vi "RudderToPoint.vi"(1 "Angle to Check":dbl) -> (8 "Goodness":dbl)   [LabVIEW 2012]
doc: "Takes in an angle to check, and returns a goodness value related to how close said angle is to the angle between the robot and the waypoint.\n\nTODO: Convert to using angle class"
uses:
  Sailbot Trunk/Software/2-Think/2 Typedefs/UTM Location.ctl
  Midbrain/Act/GoToWaypoint/RudderToPointEnum.ctl
  Utilities/Math/Angles/Angle/Angle.lvclass
panel:
  in  "Enum":T1
  in  "Robot Angle":dbl
  in  "Robot Location":T2 {"North" format="%#_10f"; "East" format="%#_8f"}
  in  "Waypoint":T2 {"North" format="%#_10f"; "East" format="%#_8f"}
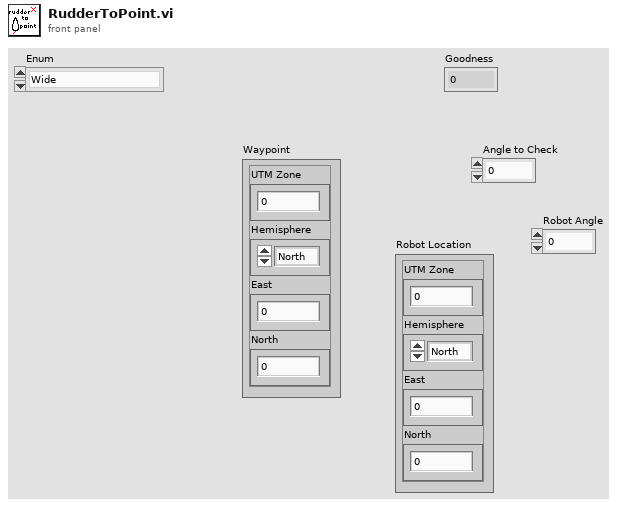
[diagram p1: front panel]
types:
  T1 = typedef "RudderToPointEnum.ctl" = enum16{"Wide", "Very Wide", "Conservative", "Narrow", "Moderate"}
  T2 = typedef "UTM Location.ctl" = cluster{"UTM Zone":dbl, "Hemisphere":enum16{"North", "South"}, "East":dbl, "North":dbl}
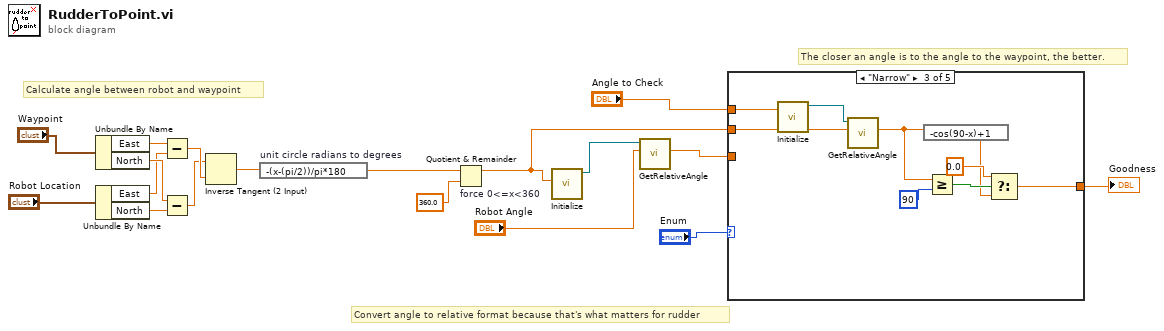
[diagram p0: block diagram]
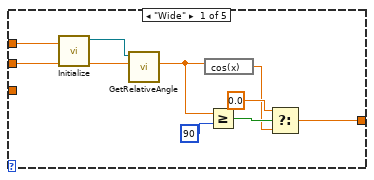
[diagram p2: hidden frame]
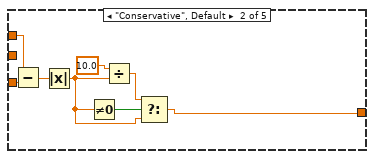
[diagram p3: hidden frame]
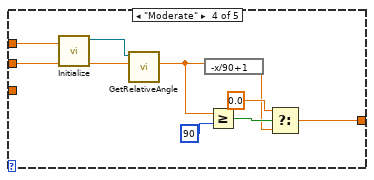
[diagram p4: hidden frame]
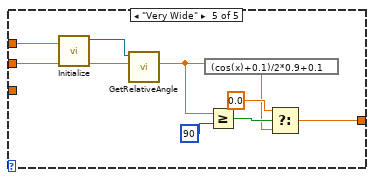
[diagram p5: hidden frame]
diagram:
  # "The closer an angle is to the angle to the waypoint, the better."
  # "Convert angle to relative format because that's what matters for rudder"
  # "Calculate angle between robot and waypoint"
  n1 = Unbundle By Name("Waypoint") -> ("East"=w13:dbl, "North"=w15:dbl)
  n2 = Unbundle By Name("Robot Location") -> ("East"=w14:dbl, "North"=w16:dbl)
  n3 = Subtract(x=w13, y=w14) -> (x-y=w18:dbl)
  n4 = Subtract(x=w15, y=w16) -> (x-y=w17:dbl)
  n5 = Inverse Tangent (2 Input) ("use inverse tangent\nto get heading")(1:w18, 2:w17) -> (0:w8:dbl)
  n6 = expression code="-(x-(pi/2))/pi*180" "unit circle radians to degrees"(w8) -> (w9:dbl)
  n7 = Quotient & Remainder "force 0<=x<360"(x=w9, y=360.0) -> (x-y*floor(x/y)=w1:dbl)  [unwired: 1 out]
  n8 = call "Initialize.vi"("Input Angle (Deg.)"=w1) -> ("Angle out"=w7:refnum<class "Angle.lvclass">)  [unwired: 9 in, 1 out]
  n9 = call "GetRelativeAngle.vi"("Boat Angle (Deg.)"="Robot Angle", "Angle in"=w7) -> ("Relative Angle"=w5:dbl)  [unwired: 8 in, 1 out]
  n10 = case shown="\"Narrow\"" "Enum" {
    tunnel: w5 -> [_ w35 _ _ _]
    tunnel: "Angle to Check" -> [w26 w34 w43 w52 w61]
    tunnel: [w19 w28 w36 w45 w54] -> w3
    tunnel: w1 -> [w27 _ w44 w53 w62]
    frame "Wide" {
      n11 = call "Initialize.vi"("Input Angle (Deg.)"=w26) -> ("Angle out"=w25:refnum<class "Angle.lvclass">)  [unwired: 9 in, 1 out]
      n12 = call "GetRelativeAngle.vi"("Boat Angle (Deg.)"=w27, "Angle in"=w25) -> ("Relative Angle"=w22:dbl)  [unwired: 8 in, 1 out]
      n13 = expression code="cos(x)"(w22) -> (w20:dbl)
      n14 = Greater Or Equal?(x=w22, y=90) -> (x >= y?=w23:bool)
      n15 = Select(t=0.0, s=w23, f=w20) -> (s? t:f=w19:dbl)
    }
    frame "Conservative", Default {
      n16 = Subtract(x=w34, y=w35) -> (x-y=w33:dbl)
      n17 = Absolute Value(x=w33) -> (abs(x)=w29:dbl)
      n18 = Not Equal To 0?(x=w29) -> (x != 0?=w31:bool)
      n19 = Divide(x=10.0, y=w29) -> (x/y=w30:dbl)
      n20 = Select(t=w30, s=w31, f=w29) -> (s? t:f=w28:dbl)
    }
    frame "Narrow" {
      n21 = call "Initialize.vi"("Input Angle (Deg.)"=w43) -> ("Angle out"=w42:refnum<class "Angle.lvclass">)  [unwired: 9 in, 1 out]
      n22 = call "GetRelativeAngle.vi"("Boat Angle (Deg.)"=w44, "Angle in"=w42) -> ("Relative Angle"=w39:dbl)  [unwired: 8 in, 1 out]
      n23 = expression code="-cos(90-x)+1"(w39) -> (w37:dbl)
      n24 = Greater Or Equal?(x=w39, y=90) -> (x >= y?=w40:bool)
      n25 = Select(t=0.0, s=w40, f=w37) -> (s? t:f=w36:dbl)
    }
    frame "Moderate" {
      n26 = call "Initialize.vi"("Input Angle (Deg.)"=w52) -> ("Angle out"=w51:refnum<class "Angle.lvclass">)  [unwired: 9 in, 1 out]
      n27 = call "GetRelativeAngle.vi"("Boat Angle (Deg.)"=w53, "Angle in"=w51) -> ("Relative Angle"=w48:dbl)  [unwired: 8 in, 1 out]
      n28 = expression code="-x/90+1"(w48) -> (w46:dbl)
      n29 = Greater Or Equal?(x=w48, y=90) -> (x >= y?=w49:bool)
      n30 = Select(t=0.0, s=w49, f=w46) -> (s? t:f=w45:dbl)
    }
    frame "Very Wide" {
      n31 = call "Initialize.vi"("Input Angle (Deg.)"=w61) -> ("Angle out"=w60:refnum<class "Angle.lvclass">)  [unwired: 9 in, 1 out]
      n32 = call "GetRelativeAngle.vi"("Boat Angle (Deg.)"=w62, "Angle in"=w60) -> ("Relative Angle"=w57:dbl)  [unwired: 8 in, 1 out]
      n33 = expression code="(cos(x)+0.1)/2*0.9+0.1"(w57) -> (w55:dbl)
      n34 = Greater Or Equal?(x=w57, y=90) -> (x >= y?=w58:bool)
      n35 = Select(t=0.0, s=w58, f=w55) -> (s? t:f=w54:dbl)
    }
  }
  "Goodness" <- w3
